vi "FGV Excel File Path.vi"(8 "Error In":errorcluster, 9 "Get/Set":enum16{"Get", "Set"}(ring), 10 "File Path Control":path) -> (0 "Error Out":errorcluster, 2 "File Path Out":path)   [LabVIEW 2015]
doc: "FGV stores excel file path."
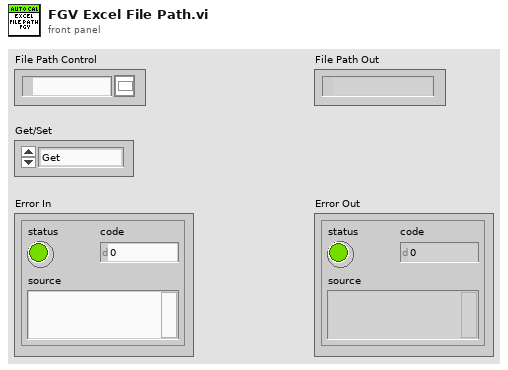
[diagram p1: front panel]
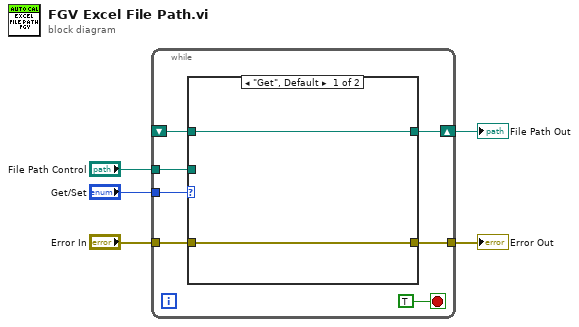
[diagram p0: block diagram]
diagram:
  n1 = while {
    tunnel: "Get/Set" -> [w12]
    tunnel: "Error In" -> [w10]
    tunnel: [w9] -> w3
    tunnel: "File Path Control" -> [w8]
    shift-right: [w7] -> w1
    shift-left: _ -> [w6]
    stop <- TRUE stop-if-true
    n2 = case shown="\"Get\", Default" w12 {
      tunnel: w10 -> [w13 w16]
      tunnel: [w13 w16] -> w9
      tunnel: w8 -> [_ w15]
      tunnel: [w14 w15] -> w7
      tunnel: w6 -> [w14 _]
      frame "Get", Default {
      }
      frame "Set" {
      }
    }
  }
  "Error Out" <- w3
  "File Path Out" <- w1
